vi "sm i32 write array and increment.vi"(9 "Identifier":string="default", 10 "value in":i32[](array[numeric]), 11 "Shared memory cluster":T1) -> (3 "Shared memory cluster output":T1)   [LabVIEW 2019, in "linuxSharedMemory.lvlib"]
uses:
  linuxSharedMemory.lvlib
  controls/sm_cluster.ctl
  <vilib>/NI/NI Linux RT IPC/Shared Memory/Pointer Operations/Write 1D Array I32.vi
  <vilib>/NI/NI Linux RT IPC/Shared Memory/Pointer Operations/In Place Write 1D Array I32.vi
  <vilib>/NI/NI Linux RT IPC/Shared Memory/Linux RT IPC.Shared Memory.lvlib
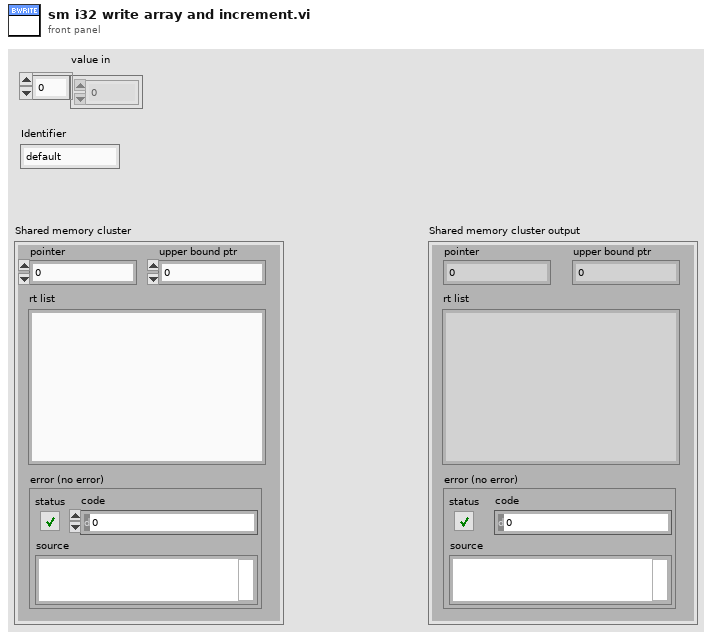
[diagram p1: front panel]
types:
  T1 = typedef "linuxSharedMemory.lvlib/sm_cluster.ctl" = cluster{"rt list":string, "error (no error)":errorcluster, "pointer":u64, "upper bound ptr":u64}
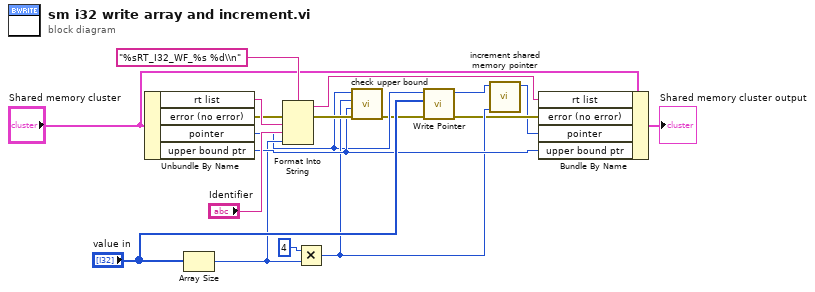
[diagram p0: block diagram]
diagram:
  n1 = Unbundle By Name("Shared memory cluster") -> ("rt list"=w14:string, "error (no error)"=w11:errorcluster, "pointer"=w4:u64, "upper bound ptr"=w7:u64)
  n2 = Array Size(array="value in") -> (size(s)=w5:i32)
  n3 = Format Into String(format string="%sRT_I32_WF_%s %d\\n", error in=w11, w14, "Identifier", w5) -> (resulting string=w13:string, error out=w10:errorcluster)  [unwired: 1 in]
  n4 = Multiply(x=4, y=w5) -> (x*y=w6:u64)
  n5 = call "check upper bound.vi"("error in (no error)"=w10, "ptr upper bound (inclusive)"=w7, "size"=w6, "ptr in"=w4) -> ("error out"=w3:errorcluster)  [unwired: 7 in]
  n6 = call-poly <vilib>:"Write Pointer.vi"("error in (no error)"=w3, "value"="value in", "pointer in"=w4) -> ("error out"=w2:errorcluster, "pointer out"=w18:u64)  [unwired: 5 in, 2 out]
  n7 = call "increment shared memory pointer.vi"("Increment value"=w6, "Shared Memory PTR in"=w18) -> ("Shared Memory PTR out"=w1:u64)  [unwired: 9 in]
  n8 = Bundle By Name(cluster="Shared memory cluster", "rt list"=w13, "error (no error)"=w2, "pointer"=w1, "upper bound ptr"=w7) -> (→"Shared memory cluster output":T1)
